vi "DSF.Engine.Memory.Cache.Transfer Group.Initialize.vi"(8 "error in (no error)":errorcluster, 10 "Device Ref in":T1=18446744073709551615 format="%.0x", 11 "Transfer Group Cache in":refnum<class "DSF.Engine.Memory.Cache.Transfer Group.lvclass">) -> (0 "error out":errorcluster, 3 "Transfer Group Cache out":refnum<class "DSF.Engine.Memory.Cache.Transfer Group.lvclass">)   [LabVIEW 2016, in "DSF.Engine.lvlib" / "DSF.Engine.Memory.Cache.Transfer Group.lvclass"]
uses:
  DSF.Engine.Memory.Cache.Transfer Group.lvclass
  <vilib>/NI Veristand/Custom Device API/Custom Device Item Ref.ctl
  DSF.Engine.Memory.Cache.Transfer Group.lvclass/DSF.Engine.Memory.Cache.Transfer Group.ctl
  DSF.Engine.Memory.Cache.Transfer.lvclass
  <vilib>/NI Veristand/Custom Device API/Custom Device API.lvlib
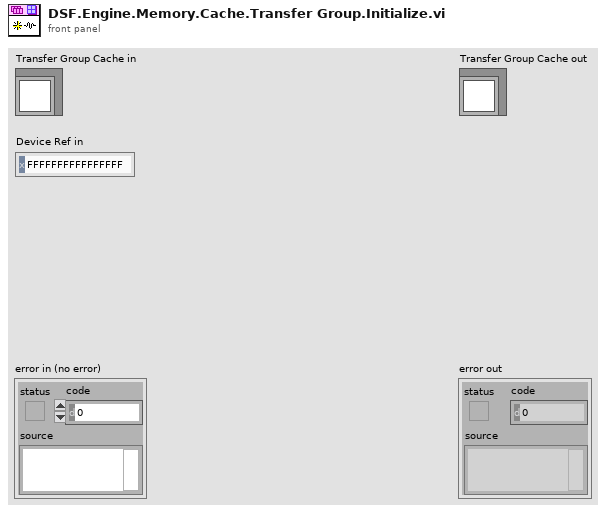
[diagram p1: front panel]
types:
  T1 = typedef "Custom Device API.lvlib/Custom Device Item Ref.ctl" = u64
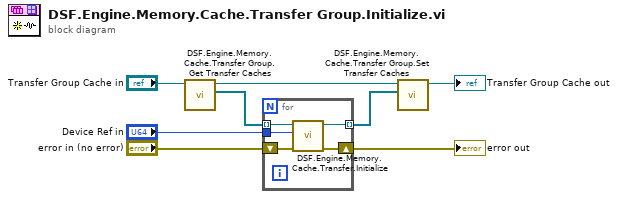
[diagram p0: block diagram]
diagram:
  n1 = call "DSF.Engine.Memory.Cache.Transfer Group.Get Transfer Caches.vi"("Transfer Group Cache in"="Transfer Group Cache in") -> ("Transfer Caches"=w6:refnum<class "DSF.Engine.Memory.Cache.Transfer.lvclass">[], "Transfer Group Cache out"=w5:refnum<class "DSF.Engine.Memory.Cache.Transfer Group.lvclass">)  [unwired: 9 in]
  n2 = for {
    tunnel: [w13] -> w7 mode=indexing
    tunnel: "Device Ref in" -> [w9]
    shift-right: [w12] -> w1
    shift-left: "error in (no error)" -> [w11]
    tunnel: w6 -> [w10] mode=indexing
    n3 = call "DSF.Engine.Memory.Cache.Transfer.Initialize.vi"("error in (no error)"=w11, "Device Ref in"=w9, "Transfer Cache in"=w10) -> ("error out"=w12:errorcluster, "Transfer Cache out"=w13:refnum<class "DSF.Engine.Memory.Cache.Transfer.lvclass">)  [unwired: 7 in]
  }
  "error out" <- w1
  n4 = call "DSF.Engine.Memory.Cache.Transfer Group.Set Transfer Caches.vi"("Transfer Caches"=w7, "Transfer Group Cache in"=w5) -> ("Transfer Group Cache out"=→"Transfer Group Cache out":refnum<class "DSF.Engine.Memory.Cache.Transfer Group.lvclass">)  [unwired: 9 in]
